vi "Slicing Engine.vi"(7 "System Parameters":T1={"Optical Parameters"={"Obj. Focal Length [mm]"=0.0, "Scan Lens EFL[mm]"=0.0, "Tube Lens EFL[mm]"=0.0, "Galvo V Range (+/-)"=0.0, "Galvo Max Half Angle [Deg]"=0.0, "Max Galvo Range[%]"=0.0}, "Vibratome"={"Z Bottom [mm]"=0.0, "Pre Cut Dwell [s]"=0.0, "Blade Frequency [RPM]"=0, "Slice Speed [mm/s]"=0.0, "Post Cut Dwell [s]"=0.0, "Ramp Time [s]"=0.0, "Start X [mm]"=0.0, "Start Y [mm]"=0.0, "Slice Length [mm]"=0.0, "Slice Axis"=enum."X Axis", "Controller VISA Ref"="COM4"}, "Table Stages"={"X Stage"={"Position"=0.0, "Is.Enabled?"=FALSE, "Is.Connected?"=FALSE, "Device SN"="45876425", "AccelerationMaximum"=50.0, "VelocityMaximum"=50.0, "Acceleration"=50.0, "Velocity"=50.0, "waitTimeout (ms)"=500000, "Model"=enum."Thorlabs LTS", "Is.Homed?"=FALSE}, "Y Stage"={"Position"=0.0, "Is.Enabled?"=FALSE, "Is.Connected?"=FALSE, "Device SN"="45995820", "AccelerationMaximum"=50.0, "VelocityMaximum"=50.0, "Acceleration"=50.0, "Velocity"=50.0, "waitTimeout (ms)"=500000, "Model"=enum."Thorlabs LTS", "Is.Homed?"=FALSE}, "Z Stage"={"Position"=0.0, "Is.Enabled?"=FALSE, "Is.Connected?"=FALSE, "Device SN"="49103464", "AccelerationMaximum"=10.0, "VelocityMaximum"=5.0, "Acceleration"=10.0, "Velocity"=5.0, "waitTimeout (ms)"=100000, "Model"=enum."None", "Is.Homed?"=FALSE}}, "Imaging Parameter"={"Raster Scan Direction"=enum."Uni Directional", "Pixel Dwell Time [Clock Cycles]"=0, "Flyback Time [Clock Cycles]"=0, "XY Center [um]"={"X"=1.0, "Y"=1.0}, "Pixel Step Size [um]"=0.0, "XY Image Size"=enum."32 x 32", "Custom"=FALSE, "Custom Size"={"X"=1, "Y"=1}, "Line Averages"=1}, "Galvo HW Parameters"={"Analog Out Channel"="GalvoCtrl/ao0,GalvoCtrl/ao1", "Min Voltage"=-10.0, "Max Voltage"=10.0, "Pixel Clock Source"="/GalvoCtrl/PFI0", "Sample Rate"=1000.0, "Line Clock Out Ch"="GalvoCtrl/port0/line0"}, "Alazar parameters"={"Trigger Settings"={"General Trigger Settings"={"Trigger Operation"=0, "Coupling ID"=2, "Range ID"=2, "Delay"=0, "Timeout Ticks"=0, "Mode"=1, "Parameter"=1}, "Trigger Engine 1"={"Trigger Engine"=0, "Source"=2, "Slope"=1, "Level"=140}, "Trigger Engine 2"={"Trigger Engine"=1000, "Source"=2048, "Slope"=2048, "Level"=140}}, "Capture Clock"={"Sample Rate"=100, "Decimation"=0, "Source"=2, "Edge"=0}, "Device ID"={"System ID"=1, "Board ID"=1}, "Ch A Input Control"={"Channel"=1, "Coupling"=2, "Range"=10, "Impedance"=2}, "Ch B Input Control"={"Channel"=2, "Coupling"=2, "Range"=10, "Impedance"=2}, "Acq Settings"={"Window Type"=1, "Record Length"=1440, "Footer"=0, "Offset"=0, "Records Per Buffer"=2048, "Samples per record"=2048, "Records Count (Records/Acq)"=2147483647, "Output Format"=10}}, "Mosaic Paramter"={"X Axis"={"Start [mm]"=0.0, "Steps [pts]"=0.0, "End [mm]"=0.0}, "Y Axis"={"Start [mm]"=0.0, "Steps [pts]"=0.0, "End [mm]"=0.0}, "Scan Pattern"=enum."Uni-directional", "Overlap Options"={"Overlap Type"=enum."No Overlap", "Percent Overlap"=0, "Justify"=enum."Start"}}, "Vibratome Axis"={"Start [mm]"=95.8, "thick[um]"=2.1, "#slices"=111}} {"Alazar parameters"."Acq Settings"."Output Format" items=["U16_LOG"=1, "U16_AMP2"=257]; "Alazar parameters"."Acq Settings"."Window Type" items=["DSP_WINDOW_NONE", "DSP_WINDOW_HANNING", "DSP_WINDOW_HAMMING", "DSP_WINDOW_BLACKMAN", "DSP_WINDOW_BLACKMAN_HARRIS", "DSP_WINDOW_BARTLETT"]; "Alazar parameters"."Acq Settings"."Footer" items=["FOOTER_NONE", "FOOTER_NPT"]; "Alazar parameters"."Ch B Input Control"."Channel" items=["A"=1, "B"=2, "C"=4, "D"=8]; "Alazar parameters"."Ch B Input Control"."Coupling" items=["AC"=1, "DC"=2]; "Alazar parameters"."Ch B Input Control"."Range" items=["20 mV"=1, "40 mV"=2, "50 mV"=3, "80 mV"=4, "100 mV"=5, "200 mV"=6, "400 mV"=7, "500 mV"=8, "800 mV"=9, "1 V"=10, "1.25 V"=33, "2 V"=11, "4 V"=12, "5 V"=13, "8 V"=14, "10 V"=15, "20 V"=16]; "Alazar parameters"."Ch B Input Control"."Impedance" items=["1 MOhm"=1, "50 Ohm"=2, ""=0]; "Alazar parameters"."Ch A Input Control"."Channel" items=["A"=1, "B"=2, "C"=4, "D"=8]; "Alazar parameters"."Ch A Input Control"."Coupling" items=["AC"=1, "DC"=2]; "Alazar parameters"."Ch A Input Control"."Range" items=["20 mV"=1, "40 mV"=2, "50 mV"=3, "80 mV"=4, "100 mV"=5, "200 mV"=6, "400 mV"=7, "500 mV"=8, "800 mV"=9, "1 V"=10, "1.25 V"=33, "2 V"=11, "4 V"=12, "5 V"=13, "8 V"=14, "10 V"=15, "20 V"=16]; "Alazar parameters"."Ch A Input Control"."Impedance" items=["1 MOhm"=1, "50 Ohm"=2, ""=0]; "Alazar parameters"."Capture Clock"."Edge" items=["Rising", "Falling"]; "Alazar parameters"."Capture Clock"."Source" items=["Internal"=1, "Fast External"=2, "Medium External"=3, "Slow External"=4, "External AC"=5, "External DC"=6, "External 10MHz"=7]; "Alazar parameters"."Trigger Settings"."General Trigger Settings"."Trigger Operation" items=["J", "K", "J OR K", "J AND K", "J XOR K", "J AND NOT K", "NOT J AND K"]; "Alazar parameters"."Trigger Settings"."General Trigger Settings"."Coupling ID" items=["AC"=1, "DC"=2]; "Alazar parameters"."Trigger Settings"."General Trigger Settings"."Range ID" items=["5 V", "1 V", "TTL"]; "Alazar parameters"."Trigger Settings"."Trigger Engine 1"."Trigger Engine" items=["J", "K"]; "Alazar parameters"."Trigger Settings"."Trigger Engine 1"."Source" items=["A", "B", "External", "Disable", "C", "D"]; "Alazar parameters"."Trigger Settings"."Trigger Engine 1"."Slope" items=["Positive"=1, "Negative"=2]; "Alazar parameters"."Trigger Settings"."Trigger Engine 2"."Trigger Engine" items=["J", "K"]; "Alazar parameters"."Trigger Settings"."Trigger Engine 2"."Source" items=["A", "B", "External", "Disable", "C", "D"]; "Alazar parameters"."Trigger Settings"."Trigger Engine 2"."Slope" items=["Positive"=1, "Negative"=2]; "Imaging Parameter"."Line Averages" min=1 max=30 step=1; "Imaging Parameter"."Flyback Time [Clock Cycles]" max=10 step=1; "Imaging Parameter"."Pixel Step Size [um]" min=0.0 max=10.0 step=0.01; "Imaging Parameter"."Custom Size"."Y" min=1 max=30 step=1; "Imaging Parameter"."Custom Size"."X" min=1 max=30 step=1; "Imaging Parameter"."XY Center [um]"."Y" min=1.0 max=30.0 step=1.0; "Imaging Parameter"."XY Center [um]"."X" min=1.0 max=30.0 step=1.0; "Imaging Parameter"."Pixel Dwell Time [Clock Cycles]" max=10 step=1}, 8 "error in (no error)":errorcluster, 10 "Action":string="Init", 11 "Last Slice?":bool) -> (0 "error out":errorcluster)   [LabVIEW 2018]
uses:
  Controls/System Parameters.ctl
  Controls/Optical Parameters.ctl
  Controls/Vibratome Parameters.ctl
  Controls/Translation Stage Parameters.ctl
  Hardware Mfg/Thorlabs Translation Stages/Controls/Translation Stage Cluster.ctl
  Controls/Translation Stage Types.ctl
  Controls/Imaging Parameters.ctl
  Controls/Scan Direction.ctl
  type defines/Alazar parameters.ctl
  Hardware Mfg/AlazarTech SDK/Controls/General Trigger Settings.ctl
  Hardware Mfg/AlazarTech SDK/Controls/Trigger Engine Controls.ctl
  Hardware Mfg/AlazarTech SDK/Controls/Clock Controls.ctl
  Hardware Mfg/AlazarTech SDK/Controls/Alazar Device ID.ctl
  Hardware Mfg/AlazarTech SDK/Controls/Channel Input Controls.ctl
  Hardware Mfg/AlazarTech SDK/Controls/Alazar Acquisition Settings.ctl
  Controls/Queue Manager Actions.ctl
  Controls/QueueNames.ctl
  Hardware Mfg/Thorlabs Translation Stages/Controls/Motion Translation Module Control.ctl
  Controls/Set Get Controls.ctl
panel:
  # "X"
  # "X"
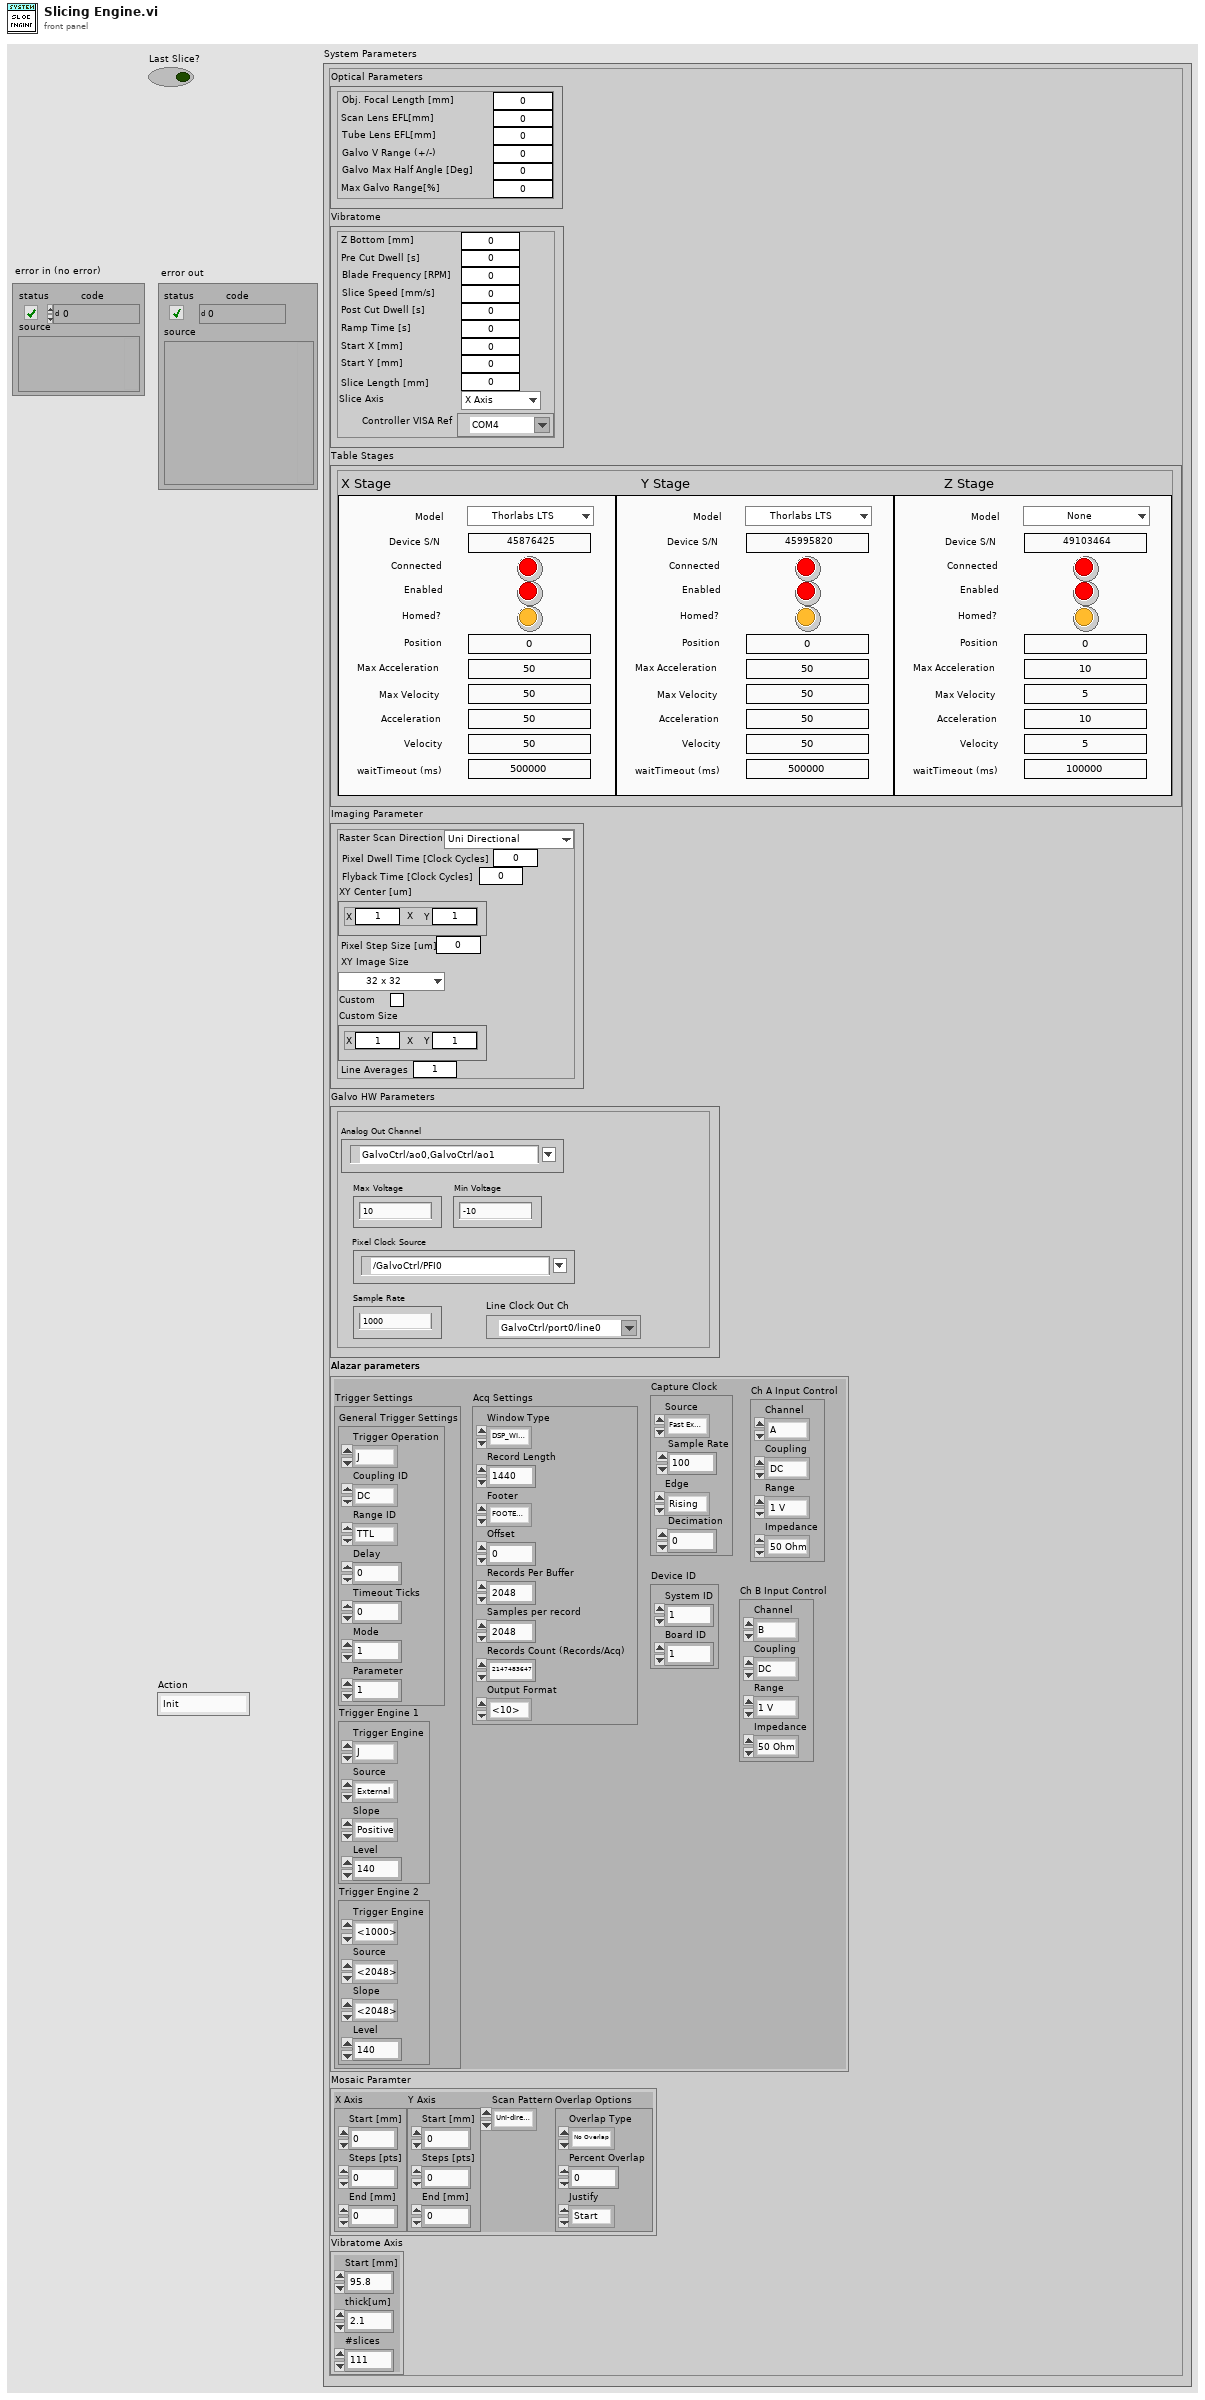
[diagram p1: front panel]
types:
  T1 = typedef "System Parameters.ctl" = cluster{"Optical Parameters":T2, "Vibratome":T3, "Table Stages":T4, "Imaging Parameter":T7, "Galvo HW Parameters":cluster{"Analog Out Channel":tag, "Min Voltage":dbl, "Max Voltage":dbl, "Pixel Clock Source":tag, "Sample Rate":dbl, "Line Clock Out Ch":tag}, "Alazar parameters":T9, "Mosaic Paramter":cluster{"X Axis":cluster{"Start [mm]":dbl, "Steps [pts]":dbl, "End [mm]":dbl}, "Y Axis":cluster{"Start [mm]":dbl, "Steps [pts]":dbl, "End [mm]":dbl}, "Scan Pattern":enum16{"Uni-directional", "Bi-Directional", "Spiral Out", "Spiral In"}, "Overlap Options":cluster{"Overlap Type":enum16{"No Overlap", "X Only", "Y Only", "X and Y"}, "Percent Overlap":u8, "Justify":enum16{"Start", "Center", "End"}}}, "Vibratome Axis":cluster{"Start [mm]":dbl, "thick[um]":dbl, "#slices":u16}}
  T2 = typedef "Optical Parameters.ctl" = cluster{"Obj. Focal Length [mm]":dbl, "Scan Lens EFL[mm]":dbl, "Tube Lens EFL[mm]":dbl, "Galvo V Range (+/-)":dbl, "Galvo Max Half Angle [Deg]":dbl, "Max Galvo Range[%]":dbl}
  T3 = typedef "Vibratome Parameters.ctl" = cluster{"Z Bottom [mm]":dbl, "Pre Cut Dwell [s]":dbl, "Blade Frequency [RPM]":u16, "Slice Speed [mm/s]":dbl, "Post Cut Dwell [s]":dbl, "Ramp Time [s]":dbl, "Start X [mm]":dbl, "Start Y [mm]":dbl, "Slice Length [mm]":dbl, "Slice Axis":enum16{"X Axis", "Y Axis", "Z Axis"}, "Controller VISA Ref":refnum<visa-resource-name>}
  T4 = typedef "Translation Stage Parameters.ctl" = cluster{"X Stage":T5, "Y Stage":T5, "Z Stage":T5}
  T5 = typedef "Translation Stage Cluster.ctl" = cluster{"Position":dbl, "Is.Enabled?":bool, "Is.Connected?":bool, "Device SN":string, "AccelerationMaximum":dbl, "VelocityMaximum":dbl, "Acceleration":dbl, "Velocity":dbl, "waitTimeout (ms)":i32, "Model":T6, "Is.Homed?":bool}
  T6 = typedef "Translation Stage Types.ctl" = enum16{"None", "Thorlabs LTS", "Thorlabs MLJ"}
  T7 = typedef "Imaging Parameters.ctl" = cluster{"Raster Scan Direction":T8, "Pixel Dwell Time [Clock Cycles]":u16, "Flyback Time [Clock Cycles]":u16, "XY Center [um]":cluster{"X":dbl, "Y":dbl}, "Pixel Step Size [um]":dbl, "XY Image Size":enum16{"32 x 32", "64 x 64", "128 x 128", "256 x 256", "512 x 512", "1024 x 1024", "2048 x 2048"}, "Custom":bool, "Custom Size":cluster{"X":u16, "Y":u16}, "Line Averages":u8}
  T8 = typedef "Scan Direction.ctl" = enum16{"Uni Directional", "Bi Directional", "None"}
  T9 = typedef "Alazar parameters.ctl" = cluster{"Trigger Settings":cluster{"General Trigger Settings":T10, "Trigger Engine 1":T11, "Trigger Engine 2":T11}, "Capture Clock":T12, "Device ID":T13, "Ch A Input Control":T14, "Ch B Input Control":T14, "Acq Settings":T15}
  T10 = typedef "General Trigger Settings.ctl" = cluster{"Trigger Operation":u32, "Coupling ID":u32, "Range ID":u32, "Delay":u32, "Timeout Ticks":u32, "Mode":u32, "Parameter":u32}
  T11 = typedef "Trigger Engine Controls.ctl" = cluster{"Trigger Engine":u32, "Source":u32, "Slope":u32, "Level":u32}
  T12 = typedef "Clock Controls.ctl" = cluster{"Sample Rate":u32, "Decimation":u32, "Source":u32, "Edge":u32}
  T13 = typedef "Alazar Device ID.ctl" = cluster{"System ID":u32, "Board ID":u32}
  T14 = typedef "Channel Input Controls.ctl" = cluster{"Channel":u8, "Coupling":u32, "Range":u32, "Impedance":u32}
  T15 = typedef "Alazar Acquisition Settings.ctl" = cluster{"Window Type":u32, "Record Length":u32, "Footer":u32, "Offset":u32, "Records Per Buffer":u32, "Samples per record":u32, "Records Count (Records/Acq)":u32, "Output Format":u32}
  T16 = typedef "QueueNames.ctl" = enum16{"Main GUI", "Main Scan Processor", "Main Processing", "Main Saving", "Main Display", "Main Table Stage GUI", "Main Table Stage Proc.", "Scan Engine", "Vibratome GUI", "Vibratome Processor", "Slice Engine"}
  T17 = typedef "Queue Manager Actions.ctl" = enum16{"Init", "Enqueue", "Enqueue All", "Preview Queue", "Dequeue", "Get Status", "Flush Queue", "Flush All Queues", "Release All Queues", "Release Queue", "Enqueue at Opposite End"}
  T18 = typedef "Set Get Controls.ctl" = enum16{"Set", "Get"}
  T19 = typedef "Motion Translation Module Control.ctl" = enum16{"Init", "Home", "Status", "Velocity/Accel", "Position", "Jog", "Stop", "Uninit", "Enable", "Disable"}
  T20 = enum16{"Set Configuration", "Get Configuration", "Enable Motor", "Disable Motor", "Get Status", "Open Session", "Close Session", "Set Limits", "Get Limits"}
  T21 = cluster{"Source for Velocity":enum16{"Interface", "Voltage (AI)", "PWM (AI)", "Current Target (AI)", "Current Target w/ Preset (AI)"}, "Mode":enum16{"Continuous", "Stepper Motor", "Analog Position Ctrl", "Encoder"}, "Target Velocity [RPM]":i16}
  T22 = typedef "MessagePacket.ctl" = cluster{"Message":string, "Parameter":variant}
  T23 = typedef "Translation Stage Quick Status.ctl" = cluster{"Is.Enabled?":bool, "Is.Connected?":bool, "Is.Homed?":bool}
  T24 = enum16{"Left Button", "Center Button", "Right Button", "Window Close"}
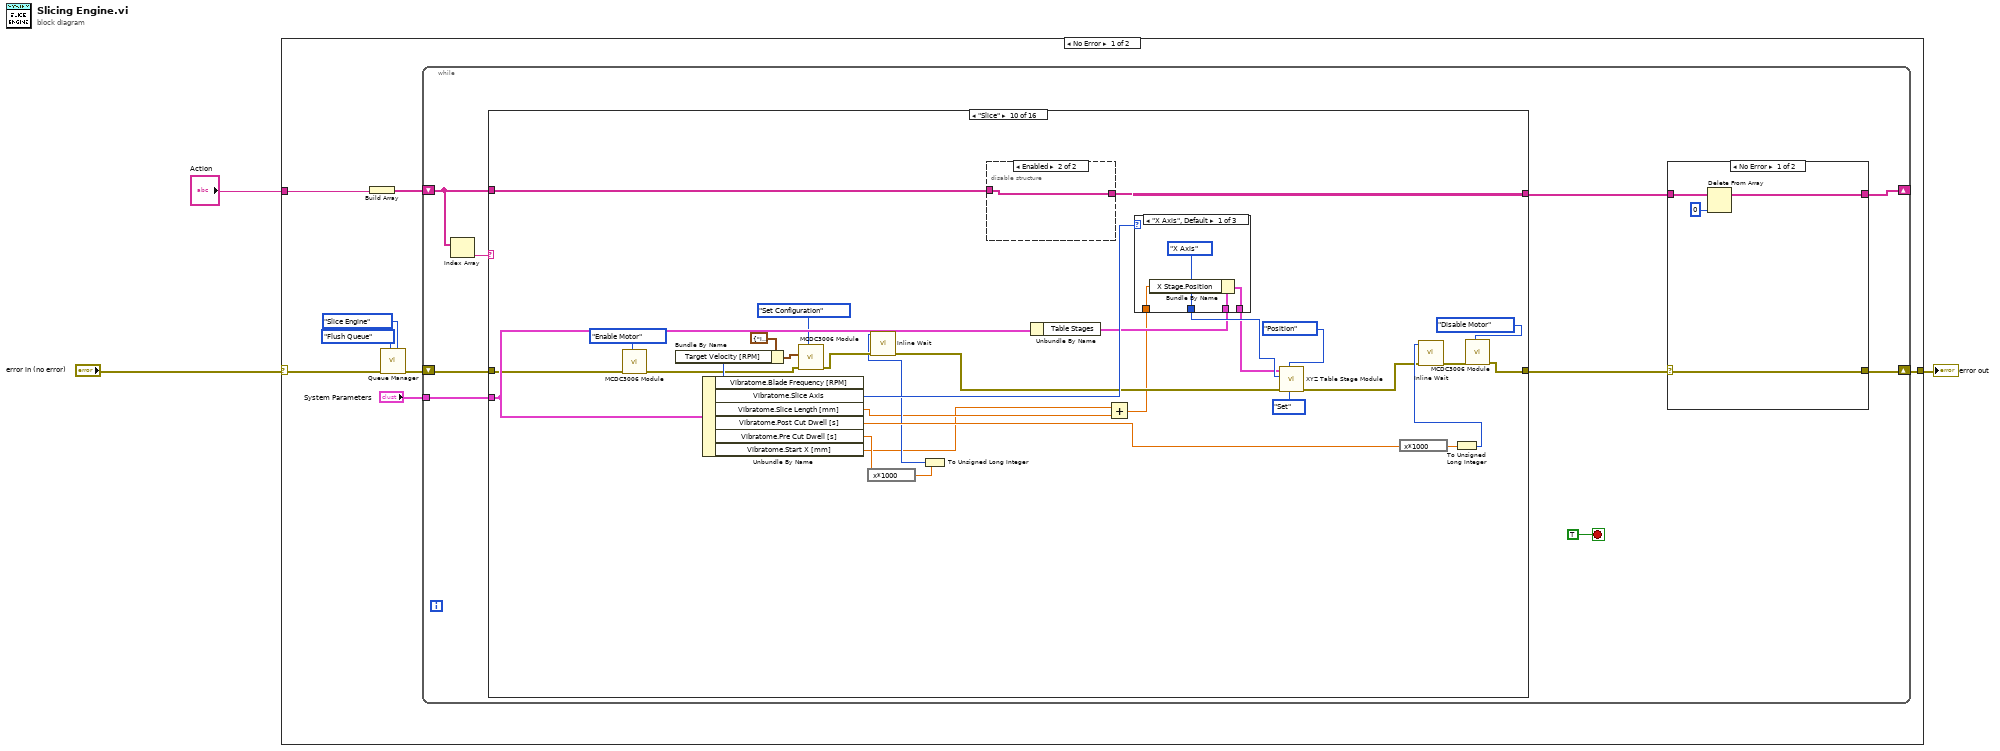
[diagram p0: block diagram]
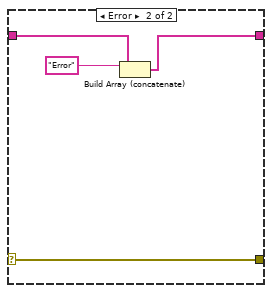
[diagram p2: hidden frame]
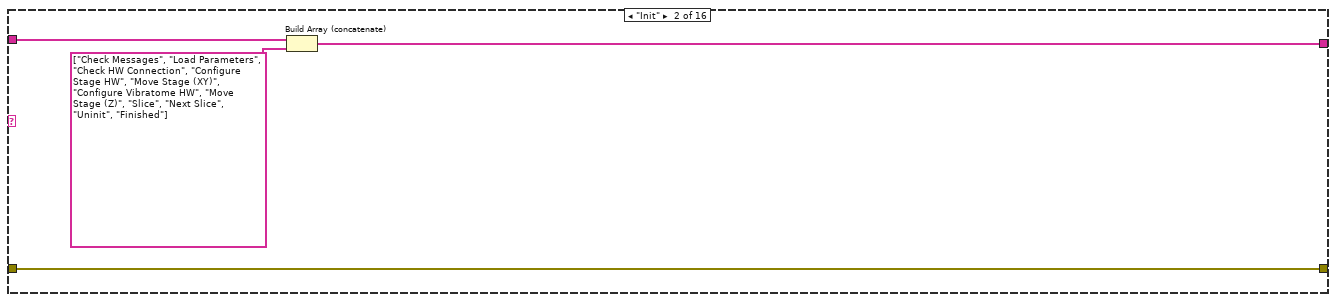
[diagram p4: hidden frame]
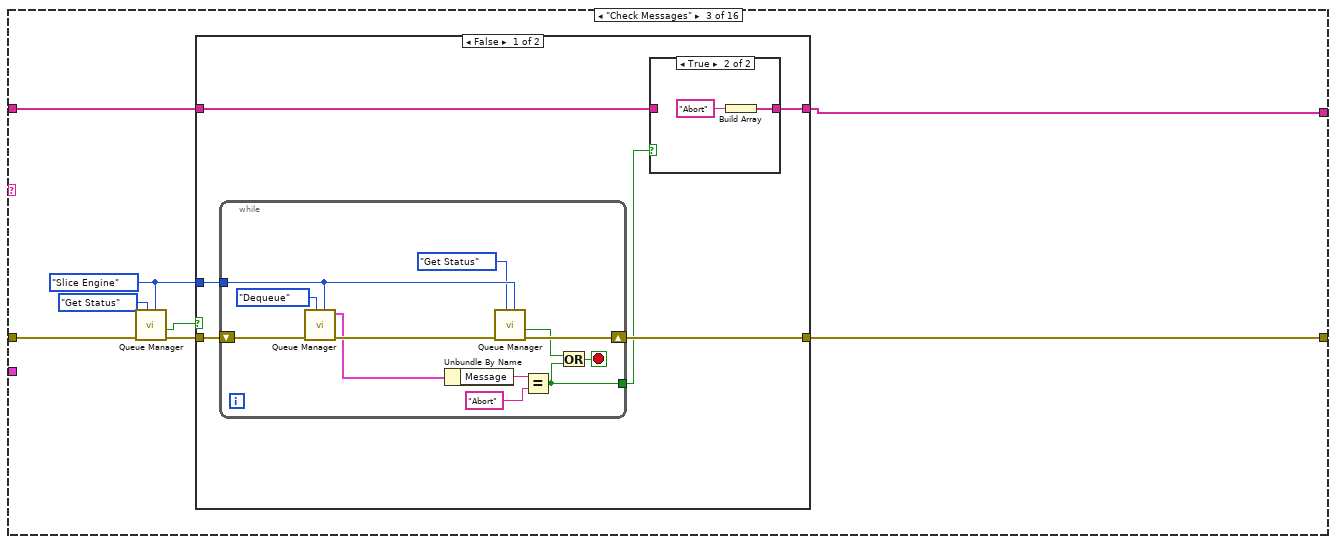
[diagram p5: hidden frame]
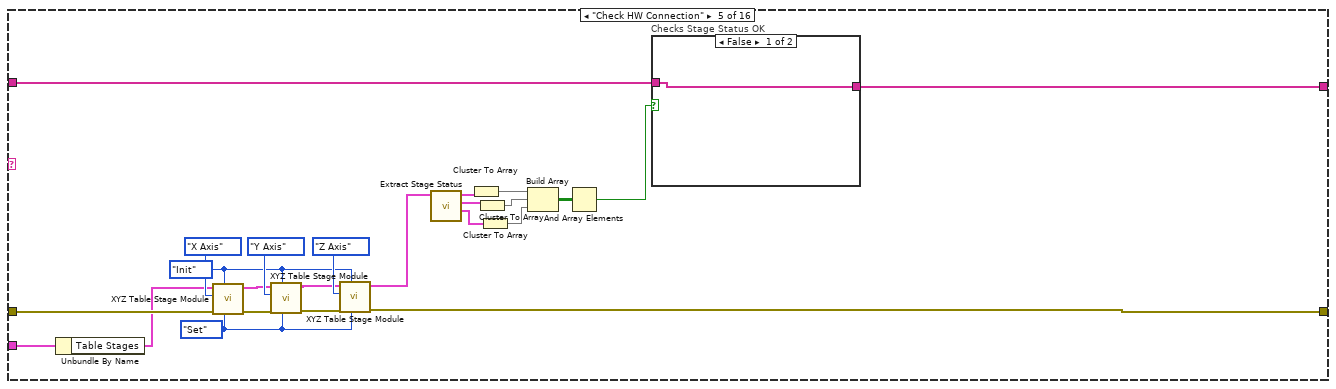
[diagram p9: hidden frame]
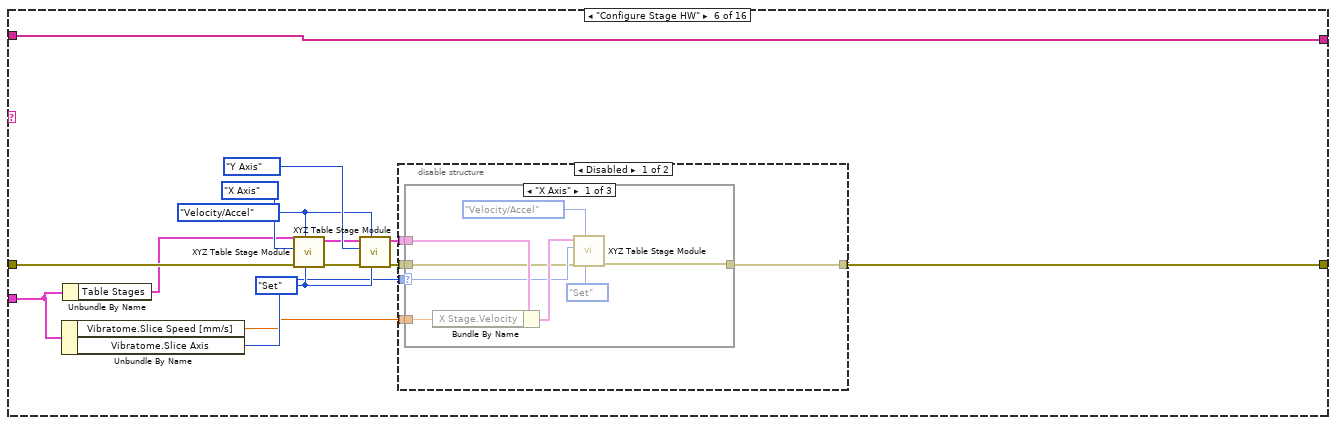
[diagram p11: hidden frame]
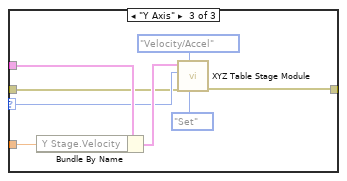
[diagram p13: hidden frame]
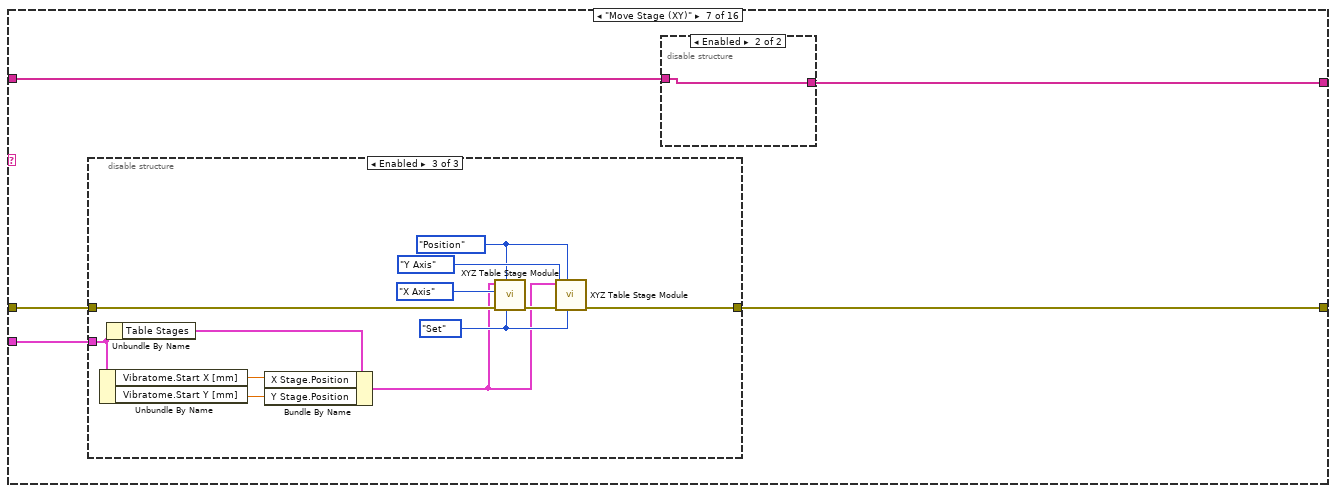
[diagram p15: hidden frame]
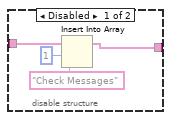
[diagram p16: hidden frame]
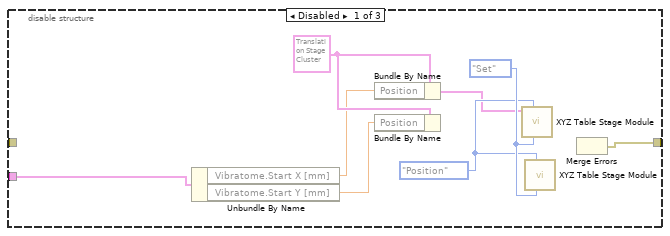
[diagram p17: hidden frame]
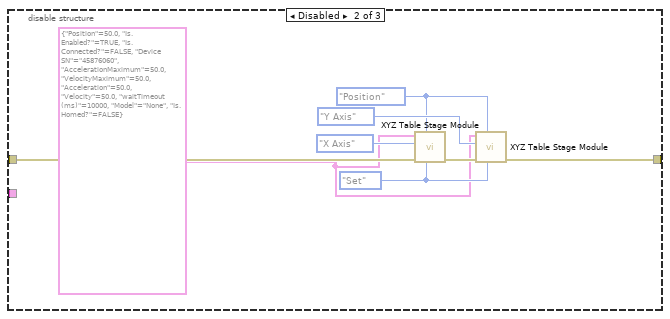
[diagram p18: hidden frame]
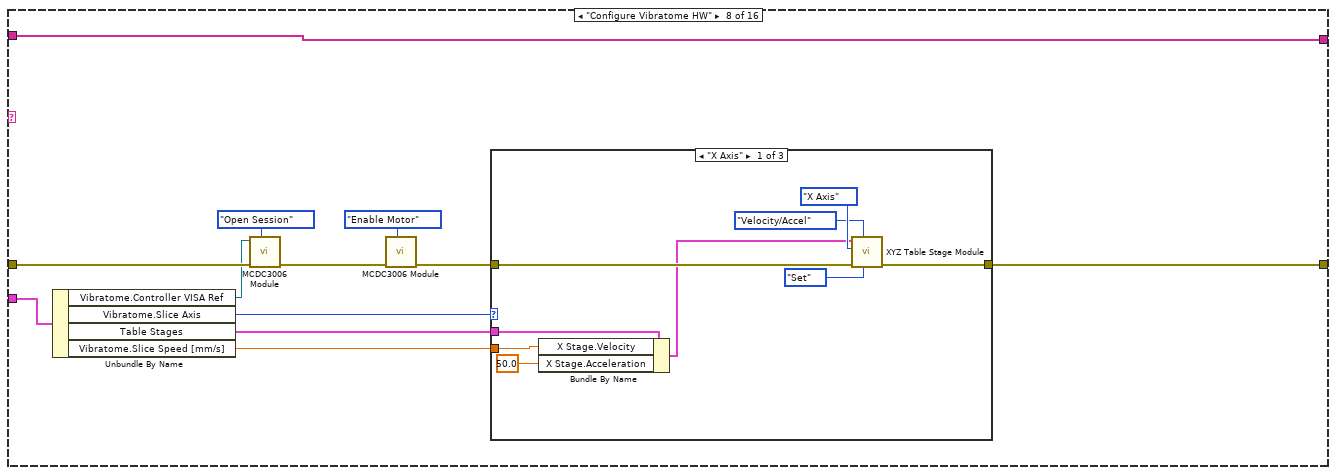
[diagram p19: hidden frame]
diagram:
  n1 = case shown="No Error" "error in (no error)" {
    selector: "error in (no error)" -> [w5 w422]
    tunnel: [w7 w422] -> w2
    tunnel: "Action" -> [w4 _]
    frame No Error {
      n2 = Build Array(w4) -> (w8:string[])
      n3 = call "Queue Manager.vi"("Queue Name"=QueueNames."Slice Engine", "Action"=Queue_Manager_Actions."Flush Queue", "Error In"=w5) -> ("Error Out"=w10:errorcluster)  [unwired: 4 in, 4 out]
      n4 = while {
        shift-right: [w15] -> _
        shift-left: w8 -> [w14]
        shift-right: [w17] -> w7
        shift-left: w10 -> [w20]
        tunnel: "System Parameters" -> [w13]
        stop <- TRUE stop-if-true
        n5 = Index Array(array=w14) -> (element=w19:string)  [unwired: 1 in]
        n6 = case shown="\"Slice\"" w19 {
          tunnel: w20 -> [w29 w31 w42 w66 w91 w107 w134 w179 w202 w247 w272 w298 w312 w316 w345 w420]
          tunnel: w14 -> [w30 w34 w36 w67 w69 w108 w136 w181 w205 w258 w273 w301 w309 w314 w346 w421]
          tunnel: [w30 w33 w35 w67 w70 w108 w135 w181 w204 w257 w273 w300 w310 w313 w346 w421] -> w16
          tunnel: [w29 w31 w37 w66 w89 w94 w133 w173 w203 w241 w274 w298 w312 w317 w343 w419] -> w18
          tunnel: w13 -> [_ _ _ _ w90 w106 w132 w180 w201 w256 w275 _ _ _ w344 _]
          frame "Unknown", Default {
          }
          frame "Init" {
            n7 = Build Array (concatenate)(w34, string[] ["Check Messages", "Load Parameters", "Check HW Connection", "Configure Stage HW", "Move Stage (XY)", "Configure Vibratome HW", "Move Stage (Z)", "Slice", "Next Slice", "Uninit", "Finished"]) -> (w33:string[])
          }
          frame "Check Messages" {
            w38 = QueueNames."Slice Engine" ("Queue Name")
            n8 = call "Queue Manager.vi"("Queue Name"=w38, "Action"=Queue_Manager_Actions."Get Status", "Error In"=w42) -> ("Error Out"=w39:errorcluster, "Empty?"=w40:bool)  [unwired: 4 in, 3 out]
            n9 = case shown="False" w40 {
              tunnel: w39 -> [w48 w64]
              tunnel: w38 -> [w47 _]
              tunnel: [w46 w64] -> w37
              tunnel: w36 -> [w44 w65]
              tunnel: [w43 w65] -> w35
              frame False {
                n10 = while {
                  tunnel: w47 -> [w59]
                  shift-right: [w60] -> w46
                  shift-left: w48 -> [w63]
                  tunnel: [w52] -> w45
                  stop <- w53 stop-if-true
                  n11 = call "Queue Manager.vi"("Queue Name"=w59, "Action"=Queue_Manager_Actions."Dequeue", "Error In"=w63) -> ("Error Out"=w61:errorcluster, "Message Packet [Out]"=w57:T22)  [unwired: 4 in, 3 out]
                  n12 = Unbundle By Name(w57) -> ("Message"=w56:string)
                  n13 = call "Queue Manager.vi"("Queue Name"=w59, "Action"=Queue_Manager_Actions."Get Status", "Error In"=w61) -> ("Error Out"=w60:errorcluster, "Empty?"=w54:bool)  [unwired: 4 in, 3 out]
                  n14 = Equal?(x=w56, y="Abort") -> (x = y?=w52:bool)
                  n15 = Or(x=w54, y=w52) -> (x .or. y?=w53:bool)
                }
                n16 = case shown="True" w45 {
                  tunnel: w44 -> [w49 _]
                  tunnel: [w49 w50] -> w43
                  frame False {
                  }
                  frame True {
                    n17 = Build Array("Abort") -> (w50:string[])
                  }
                }
              }
              frame True {
              }
            }
          }
          frame "Load Parameters" {
          }
          frame "Check HW Connection" {
            w82 = Set_Get_Controls."Set" ("Set/Get")
            w83 = Motion_Translation_Module_Control."Init" ("Action")
            n18 = Unbundle By Name(w90) -> ("Table Stages"=w81:T4)
            n19 = call "XYZ Table Stage Module.vi"("Set/Get"=w82, "Action"=w83, "Error In"=w91, "Axis"=enum16{"X Axis", "Y Axis", "Z Axis"}."X Axis", "Table Stages"=w81) -> ("Error Out"=w88:errorcluster, "Table Stages [out]"=w80:T4)  [unwired: 5 in]
            n20 = call "XYZ Table Stage Module.vi"("Set/Get"=w82, "Action"=w83, "Error In"=w88, "Axis"=enum16{"X Axis", "Y Axis", "Z Axis"}."Y Axis", "Table Stages"=w80) -> ("Error Out"=w87:errorcluster, "Table Stages [out]"=w79:T4)  [unwired: 5 in]
            n21 = call "XYZ Table Stage Module.vi"("Set/Get"=w82, "Action"=w83, "Error In"=w87, "Axis"=enum16{"X Axis", "Y Axis", "Z Axis"}."Z Axis", "Table Stages"=w79) -> ("Error Out"=w89:errorcluster, "Table Stages [out]"=w78:T4)  [unwired: 5 in]
            n22 = call "Extract Stage Status.vi"("Table Stages"=w78) -> ("Z Stage"=w75:T23, "Y Stage"=w76:T23, "X Stage"=w77:T23)  [unwired: 8 in]
            n23 = Cluster To Array(cluster=w77) -> (array=w74:bool[])
            n24 = Cluster To Array(cluster=w76) -> (array=w73:bool[])
            n25 = Cluster To Array(cluster=w75) -> (array=w72:bool[])
            n26 = Build Array(w74, w73, w72) -> (w71:bool[][])
            n27 = And Array Elements(Boolean array=w71) -> (logical AND=w68:bool)
            n28 = case "Checks Stage Status OK" shown="False" w68 {
              tunnel: [w92 w93] -> w70
              tunnel: w69 -> [w92 w93]
              frame False {
              }
              frame True {
              }
            }
          }
          frame "Configure Stage HW" {
            w101 = Set_Get_Controls."Set" ("Set/Get")
            w102 = Motion_Translation_Module_Control."Velocity/Accel" ("Action")
            n29 = Unbundle By Name(w106) -> ("Vibratome.Slice Speed [mm/s]"=w97:dbl, "Vibratome.Slice Axis"=w98:enum16{"X Axis", "Y Axis", "Z Axis"})
            n30 = Unbundle By Name(w106) -> ("Table Stages"=w99:T4)
            n31 = call "XYZ Table Stage Module.vi"("Set/Get"=w101, "Action"=w102, "Error In"=w107, "Axis"=enum16{"X Axis", "Y Axis", "Z Axis"}."X Axis", "Table Stages"=w99) -> ("Error Out"=w105:errorcluster, "Table Stages [out]"=w100:T4)  [unwired: 5 in]
            n32 = call "XYZ Table Stage Module.vi"("Set/Get"=w101, "Action"=w102, "Error In"=w105, "Axis"=enum16{"X Axis", "Y Axis", "Z Axis"}."Y Axis", "Table Stages"=w100) -> ("Error Out"=w95:errorcluster, "Table Stages [out]"=w96:T4)  [unwired: 5 in]
            n33 = disable-structure shown="Disabled" {
              disable-tunnel: w98 -> [w113 _]
              disable-tunnel: w97 -> [w112 _]
              disable-tunnel: w96 -> [w111 _]
              disable-tunnel: w95 -> [w110 w131]
              disable-tunnel: [w109 w131] -> w94
              frame Disabled {
                n34 = case shown="\"X Axis\"" w113 {
                  selector: w113 -> [w118 _ w127]
                  tunnel: w112 -> [w121 _ w130]
                  tunnel: w111 -> [w120 _ w129]
                  tunnel: w110 -> [w117 w122 w126]
                  tunnel: [w116 w122 w125] -> w109
                  frame "X Axis" {
                    n35 = Bundle By Name(cluster=w120, "X Stage.Velocity"=w121) -> (w119:T4)
                    n36 = call "XYZ Table Stage Module.vi"("Set/Get"=Set_Get_Controls."Set", "Action"=Motion_Translation_Module_Control."Velocity/Accel", "Error In"=w117, "Axis"=w118, "Table Stages"=w119) -> ("Error Out"=w116:errorcluster)  [unwired: 5 in, 1 out]
                  }
                  frame "Z Axis" {
                  }
                  frame "Y Axis" {
                    n37 = Bundle By Name(cluster=w129, "Y Stage.Velocity"=w130) -> (w128:T4)
                    n38 = call "XYZ Table Stage Module.vi"("Set/Get"=Set_Get_Controls."Set", "Action"=Motion_Translation_Module_Control."Velocity/Accel", "Error In"=w126, "Axis"=w127, "Table Stages"=w128) -> ("Error Out"=w125:errorcluster)  [unwired: 5 in, 1 out]
                  }
                }
              }
              frame Enabled {
              }
            }
          }
          frame "Move Stage (XY)" {
            n39 = disable-structure shown="Enabled" {
              disable-tunnel: w134 -> [_ w155 w167]
              disable-tunnel: [w149 w156 w168] -> w133
              disable-tunnel: w132 -> [w147 _ w162]
              frame Disabled {
                w148 = T5 {"Position"=0.0, "Is.Enabled?"=TRUE, "Is.Connected?"=FALSE, "Device SN"="45876060", "AccelerationMaximum"=50.0, "VelocityMaximum"=50.0, "Acceleration"=50.0, "Velocity"=50.0, "waitTimeout (ms)"=10000, "Model"=enum."None", "Is.Homed?"=FALSE} ("Cluster In")
                w143 = Motion_Translation_Module_Control."Position" ("Action")
                w144 = Set_Get_Controls."Set" ("Set/Get")
                n40 = Unbundle By Name(w147) -> ("Vibratome.Start X [mm]"=w146:dbl, "Vibratome.Start Y [mm]"=w145:dbl)
                n41 = Bundle By Name(cluster=w148, "Position"=w146) -> (w142:T5)
                n42 = Bundle By Name(cluster=w148, "Position"=w145) -> ()  [unwired: 1 out]
                n43 = call "XYZ Table Stage Module.vi"("Set/Get"=w144, "Action"=w143, "Table Stages"=w142) -> ()  [unwired: 7 in, 2 out]
                n44 = call "XYZ Table Stage Module.vi"("Set/Get"=w144, "Action"=w143) -> ()  [unwired: 8 in, 2 out]
                n45 = Merge Errors() -> (w149:errorcluster)  [unwired: 2 in]
              }
              frame Disabled {
                w151 = Set_Get_Controls."Set" ("Set/Get")
                w152 = Motion_Translation_Module_Control."Position" ("Action")
                w150 = T5 {"Position"=50.0, "Is.Enabled?"=TRUE, "Is.Connected?"=FALSE, "Device SN"="45876060", "AccelerationMaximum"=50.0, "VelocityMaximum"=50.0, "Acceleration"=50.0, "Velocity"=50.0, "waitTimeout (ms)"=10000, "Model"=enum."None", "Is.Homed?"=FALSE} ("Cluster In")
                n46 = call "XYZ Table Stage Module.vi"("Set/Get"=w151, "Action"=w152, "Error In"=w155, "Axis"=enum16{"X Axis", "Y Axis", "Z Axis"}."X Axis", "Table Stages"=w150) -> ("Error Out"=w157:errorcluster)  [unwired: 5 in, 1 out]
                n47 = call "XYZ Table Stage Module.vi"("Set/Get"=w151, "Action"=w152, "Error In"=w157, "Axis"=enum16{"X Axis", "Y Axis", "Z Axis"}."Y Axis", "Table Stages"=w150) -> ("Error Out"=w156:errorcluster)  [unwired: 5 in, 1 out]
              }
              frame Enabled {
                w163 = Set_Get_Controls."Set" ("Set/Get")
                w164 = Motion_Translation_Module_Control."Position" ("Action")
                n48 = Unbundle By Name(w162) -> ("Vibratome.Start X [mm]"=w160:dbl, "Vibratome.Start Y [mm]"=w159:dbl)
                n49 = Unbundle By Name(w162) -> ("Table Stages"=w161:T4)
                n50 = Bundle By Name(cluster=w161, "X Stage.Position"=w160, "Y Stage.Position"=w159) -> (w158:T4)
                n51 = call "XYZ Table Stage Module.vi"("Set/Get"=w163, "Action"=w164, "Error In"=w167, "Axis"=enum16{"X Axis", "Y Axis", "Z Axis"}."X Axis", "Table Stages"=w158) -> ("Error Out"=w169:errorcluster)  [unwired: 5 in, 1 out]
                n52 = call "XYZ Table Stage Module.vi"("Set/Get"=w163, "Action"=w164, "Error In"=w169, "Axis"=enum16{"X Axis", "Y Axis", "Z Axis"}."Y Axis", "Table Stages"=w158) -> ("Error Out"=w168:errorcluster)  [unwired: 5 in, 1 out]
              }
            }
            n53 = disable-structure shown="Enabled" {
              disable-tunnel: w136 -> [w140 w141]
              disable-tunnel: [w139 w141] -> w135
              frame Disabled {
                n54 = Insert Into Array(array=w140, index=1, new element="Check Messages" ("new element/subarray")) -> (w139:string[])
              }
              frame Enabled {
              }
            }
          }
          frame "Configure Vibratome HW" {
            n55 = Unbundle By Name(w180) -> ("Vibratome.Controller VISA Ref"=w177:refnum<visa-resource-name>, "Vibratome.Slice Axis"=w172:enum16{"X Axis", "Y Axis", "Z Axis"}, "Table Stages"=w170:T4, "Vibratome.Slice Speed [mm/s]"=w171:dbl)
            n56 = call "MCDC3006 Module.vi"("Actions"=T20."Open Session", "Error In"=w179, "VISA resource name"=w177) -> ("Error Out"=w175:errorcluster)  [unwired: 4 in, 4 out]
            n57 = call "MCDC3006 Module.vi"("Actions"=T20."Enable Motor", "Error In"=w175) -> ("Error Out"=w174:errorcluster)  [unwired: 5 in, 4 out]
            n58 = case shown="\"X Axis\"" w172 {
              tunnel: [w190 w191 w200] -> w173
              tunnel: w174 -> [w185 w191 w196]
              tunnel: w171 -> [w186 _ w195]
              tunnel: w170 -> [w183 _ w194]
              frame "X Axis" {
                n59 = Bundle By Name(cluster=w183, "X Stage.Velocity"=w186, "X Stage.Acceleration"=50.0 ("Acceleration")) -> (w182:T4)
                n60 = call "XYZ Table Stage Module.vi"("Set/Get"=Set_Get_Controls."Set", "Action"=Motion_Translation_Module_Control."Velocity/Accel", "Error In"=w185, "Axis"=enum16{"X Axis", "Y Axis", "Z Axis"}."X Axis", "Table Stages"=w182) -> ("Error Out"=w190:errorcluster)  [unwired: 5 in, 1 out]
              }
              frame "Z Axis" {
              }
              frame "Y Axis" {
                n61 = Bundle By Name(cluster=w194, "Y Stage.Velocity"=w195, "Y Stage.Acceleration"=50.0 ("Acceleration")) -> (w192:T4)
                n62 = call "XYZ Table Stage Module.vi"("Set/Get"=Set_Get_Controls."Set", "Action"=Motion_Translation_Module_Control."Velocity/Accel", "Error In"=w196, "Axis"=enum16{"X Axis", "Y Axis", "Z Axis"}."Y Axis", "Table Stages"=w192) -> ("Error Out"=w200:errorcluster)  [unwired: 5 in, 1 out]
              }
            }
          }
          frame "Move Stage (Z)" {
            n63 = disable-structure shown="Disabled" {
              disable-tunnel: [w214 w222] -> w203
              disable-tunnel: w202 -> [w213 w222]
              disable-tunnel: w201 -> [w212 _]
              frame Disabled {
                n64 = Unbundle By Name(w212) -> ("Table Stages"=w211:T4)
                n65 = call "XYZ Table Stage Module.vi"("Set/Get"=Set_Get_Controls."Get", "Action"=Motion_Translation_Module_Control."Position", "Error In"=w213, "Axis"=enum16{"X Axis", "Y Axis", "Z Axis"}."Z Axis", "Table Stages"=w211) -> ("Error Out"=w215:errorcluster, "Table Stages [out]"=w210:T4)  [unwired: 5 in]
                n66 = Unbundle By Name(w210) -> ("Z Stage.Position"=w208:dbl)
                n67 = Add(x=w208, y=0.2) -> (x+y=w206:dbl)
                n68 = Bundle By Name(cluster=w210, "Z Stage.Position"=w206) -> (w209:T4)
                n69 = call "XYZ Table Stage Module.vi"("Set/Get"=Set_Get_Controls."Set", "Action"=Motion_Translation_Module_Control."Position", "Error In"=w215, "Axis"=enum16{"X Axis", "Y Axis", "Z Axis"}."Z Axis", "Table Stages"=w209) -> ("Error Out"=w214:errorcluster)  [unwired: 5 in, 1 out]
              }
              frame Enabled {
              }
            }
            n70 = disable-structure shown="Enabled" {
              disable-tunnel: w205 -> [w226 w227]
              disable-tunnel: [w225 w227] -> w204
              frame Disabled {
                n71 = Insert Into Array(array=w226, index=1, new element="Check Messages" ("new element/subarray")) -> (w225:string[])
              }
              frame Enabled {
              }
            }
          }
          frame "Slice" {
            n72 = call "MCDC3006 Module.vi"("Actions"=T20."Enable Motor", "Error In"=w247) -> ("Error Out"=w246:errorcluster)  [unwired: 5 in, 4 out]
            n73 = Unbundle By Name(w256) -> ("Vibratome.Blade Frequency [RPM]"=w251:u16, "Vibratome.Slice Axis"=w255:enum16{"X Axis", "Y Axis", "Z Axis"}, "Vibratome.Slice Length [mm]"=w235:dbl, "Vibratome.Post Cut Dwell [s]"=w249:dbl, "Vibratome.Pre Cut Dwell [s]"=w245:dbl, "Vibratome.Start X [mm]"=w234:dbl)
            n74 = Bundle By Name(cluster=T21 {"Source for Velocity"=enum."Interface", "Mode"=enum."Continuous", "Target Velocity [RPM]"=0} ("Configuration [In]"), "Target Velocity [RPM]"=w251) -> (w250:T21)
            n75 = call "MCDC3006 Module.vi"("Actions"=T20."Set Configuration", "Error In"=w246, "Configuration [In]"=w250) -> ("Error Out"=w254:errorcluster)  [unwired: 4 in, 4 out]
            n76 = expression code="x*1000"(w245) -> (w244:dbl)
            n77 = To Unsigned Long Integer(number=w244) -> (unsigned 32bit integer=w243:u32)
            n78 = call "Inline Wait.vi"("Error In"=w254, "milliseconds to wait"=w243) -> ("Error Out"=w236:errorcluster)  [unwired: 9 in]
            n79 = disable-structure shown="Enabled" {
              disable-tunnel: w258 -> [w270 w271]
              disable-tunnel: [w269 w271] -> w257
              frame Disabled {
                n80 = Insert Into Array(array=w270, index=1, new element="Check Messages" ("new element/subarray")) -> (w269:string[])
              }
              frame Enabled {
              }
            }
            n81 = Unbundle By Name(w256) -> ("Table Stages"=w231:T4)
            n82 = Add(x=w234, y=w235) -> (x+y=w230:dbl)
            n83 = case shown="\"X Axis\", Default" w255 {
              tunnel: [enum16{"X Axis", "Y Axis", "Z Axis"}."X Axis" ("Axis") _ enum16{"X Axis", "Y Axis", "Z Axis"}."Y Axis" ("Axis")] -> w232
              tunnel: w231 -> [w261 _ w264]
              tunnel: w230 -> [w260 _ w265]
              tunnel: [w259 _ w263] -> w229
              frame "X Axis", Default {
                n84 = Bundle By Name(cluster=w261, "X Stage.Position"=w260) -> (w259:T4)
              }
              frame "Z Axis" {
              }
              frame "Y Axis" {
                n85 = Bundle By Name(cluster=w264, "X Stage.Position"=w265) -> (w263:T4)
              }
            }
            n86 = call "XYZ Table Stage Module.vi"("Set/Get"=Set_Get_Controls."Set", "Action"=Motion_Translation_Module_Control."Position", "Error In"=w236, "Axis"=w232, "Table Stages"=w229) -> ("Error Out"=w233:errorcluster)  [unwired: 5 in, 1 out]
            n87 = expression code="x*1000"(w249) -> (w240:dbl)
            n88 = To Unsigned Long Integer(number=w240) -> (unsigned 32bit integer=w239:u32)
            n89 = call "Inline Wait.vi"("Error In"=w233, "milliseconds to wait"=w239) -> ("Error Out"=w242:errorcluster)  [unwired: 9 in]
            n90 = call "MCDC3006 Module.vi"("Actions"=T20."Disable Motor", "Error In"=w242) -> ("Error Out"=w241:errorcluster)  [unwired: 5 in, 4 out]
          }
          frame "set slice speed" {
            n91 = Unbundle By Name(w275) -> ("Vibratome.Slice Axis"=w278:enum16{"X Axis", "Y Axis", "Z Axis"}, "Table Stages"=w276:T4, "Vibratome.Slice Speed [mm/s]"=w277:dbl)
            n92 = case shown="\"X Axis\"" w278 {
              tunnel: [w287 w288 w297] -> w274
              tunnel: w272 -> [w282 w288 w293]
              tunnel: w277 -> [w283 _ w292]
              tunnel: w276 -> [w280 _ w291]
              frame "X Axis" {
                n93 = Bundle By Name(cluster=w280, "X Stage.Velocity"=w283, "X Stage.Acceleration"=50.0 ("Acceleration")) -> (w279:T4)
                n94 = call "XYZ Table Stage Module.vi"("Set/Get"=Set_Get_Controls."Set", "Action"=Motion_Translation_Module_Control."Velocity/Accel", "Error In"=w282, "Axis"=enum16{"X Axis", "Y Axis", "Z Axis"}."X Axis", "Table Stages"=w279) -> ("Error Out"=w287:errorcluster)  [unwired: 5 in, 1 out]
              }
              frame "Z Axis" {
              }
              frame "Y Axis" {
                n95 = Bundle By Name(cluster=w291, "Y Stage.Velocity"=w292, "Y Stage.Acceleration"=50.0 ("Acceleration")) -> (w289:T4)
                n96 = call "XYZ Table Stage Module.vi"("Set/Get"=Set_Get_Controls."Set", "Action"=Motion_Translation_Module_Control."Velocity/Accel", "Error In"=w293, "Axis"=enum16{"X Axis", "Y Axis", "Z Axis"}."Y Axis", "Table Stages"=w289) -> ("Error Out"=w297:errorcluster)  [unwired: 5 in, 1 out]
              }
            }
          }
          frame "Next Slice" {
            n97 = case shown="False" "Last Slice?" {
              tunnel: w301 -> [w305 w306]
              tunnel: [w304 w306] -> w300
              frame False {
                n98 = Insert Into Array(array=w305, index=1, new element=string[] ["Move Stage (Z)", "set slice speed", "Slice", "Next Slice"]) -> (w304:string[])
              }
              frame True {
              }
            }
          }
          frame "Abort" {
            n99 = Insert Into Array(array=w309, index=1, new element #1="Uninit", new element #2="Finished") -> (w310:string[])
          }
          frame "Error" {
            n100 = control-ref of="This VI"() -> (w327:refnum<vi>)
            n101 = property class="VI"(reference=w327) -> ("Name"=w330:string, "Callers"=w332:string[])  [unwired: 1 in, 2 out]
            n102 = Unbundle(w316) -> ("code"=w326:i32, "source"=w325:string)  [unwired: 1 out]
            n103 = Array To Spreadsheet String(delimiter (Tab)=">", array=w332, 3:"%s" ("format string")) -> (spreadsheet string=w331:string)
            n104 = Format Into String(format string="VI Name: %s\nCallers: %s\nError Code: %d\nError Message: %s", initial string="The following error occurred:\n" ("message"), w330, w331, w326, w325) -> (resulting string=w324:string, error out=w318:errorcluster)  [unwired: 1 in]
            n105 = call <vilib>:"Clear Errors.vi"("error in (no error)"=w318) -> ()  [unwired: 5 in, 2 out]
            n106 = call <vilib>:"Three Button Dialog.vi"("Allow user to close window? (TRUE)"=FALSE, "Window Title (\"\")"="Error" ("Window Title (\"\")"), "Right Button Text (\"Cancel\")"="Abort" ("Right Button Text (\"Cancel\")"), "Center Button Text (\"No\")"="Retry" ("Center Button Text (\"No\")"), "Left Button Text (\"Yes\")"="Continue" ("Left Button Text (\"Yes\")"), "message"=w324) -> ("Which Button?"=w315:T24)  [unwired: 5 in]
            n107 = case shown="\"Right Button\"" w315 {
              tunnel: w314 -> [w337 w341 w342]
              tunnel: [w336 w340 w342] -> w313
              frame "Left Button", Default {
                # "Continue"
                n108 = Delete From Array(array=w337, index=0) -> (array with subset deleted=w336:string[])  [unwired: 1 in, 1 out]
              }
              frame "Right Button" {
                # "Abort"
                n109 = Insert Into Array(array=w341, index=1, new element="Abort") -> (w340:string[])
              }
              frame "Center Button" {
                # "Retry"
              }
            }
            n110 = call <vilib>:"Clear Errors.vi"("error in (no error)"=w316) -> ("error out"=w317:errorcluster)  [unwired: 5 in, 1 out]
          }
          frame "Uninit" {
            n111 = disable-structure shown="Enabled" {
              disable-tunnel: w345 -> [w350 w417]
              disable-tunnel: w344 -> [w349 _]
              disable-tunnel: [w348 w410] -> w343
              frame Enabled {
                n112 = for {
                  N: 4 -> [_]
                  tunnel: [w356] -> w351 mode=indexing
                  tunnel: Motion_Translation_Module_Control."Uninit" ("Action") -> [w355]
                  tunnel: w350 -> [w354]
                  tunnel: w349 -> [w353]
                  i -> [w357]
                  n113 = case shown="0, Default" w357 {
                    tunnel: [w363 w377 w391 w403] -> w356
                    tunnel: w354 -> [w362 w376 w390 w404]
                    tunnel: w355 -> [w361 w375 w389 _]
                    tunnel: w353 -> [w360 w374 w388 _]
                    frame 0, Default {
                      # "X Stage"
                      n114 = Unbundle By Name(w360) -> ("Table Stages.X Stage.Model"=w359:T6, "Table Stages.X Stage.Device SN"=w358:string)
                      n115 = case shown="\"Thorlabs LTS\"" w359 {
                        tunnel: [w364 w371] -> w363
                        tunnel: w362 -> [w364 w370]
                        tunnel: w361 -> [_ w369]
                        tunnel: w358 -> [_ w367]
                        frame "None", Default {
                        }
                        frame "Thorlabs LTS" {
                          n116 = Bundle By Name(cluster=T5 {"Position"=0.0, "Is.Enabled?"=TRUE, "Is.Connected?"=FALSE, "Device SN"="45876539", "AccelerationMaximum"=0.0, "VelocityMaximum"=0.0, "Acceleration"=0.0, "Velocity"=0.0, "waitTimeout (ms)"=0, "Model"=enum."Thorlabs LTS", "Is.Homed?"=FALSE} ("Cluster In"), "Device SN"=w367) -> (w366:T5)
                          n117 = call "Thorlabs LTS - X Stage Module.vi"("Set/Get"=Set_Get_Controls."Set", "Error In"=w370, "Action"=w369, "Cluster In"=w366) -> ("Error Out"=w371:errorcluster)  [unwired: 6 in, 1 out]
                        }
                      }
                    }
                    frame 1 {
                      # "Y Stage"
                      n118 = Unbundle By Name(w374) -> ("Table Stages.Y Stage.Model"=w373:T6, "Table Stages.Y Stage.Device SN"=w372:string)
                      n119 = case shown="\"Thorlabs LTS\"" w373 {
                        tunnel: [w378 w385] -> w377
                        tunnel: w376 -> [w378 w384]
                        tunnel: w375 -> [_ w383]
                        tunnel: w372 -> [_ w381]
                        frame "None", Default {
                        }
                        frame "Thorlabs LTS" {
                          n120 = Bundle By Name(cluster=T5 {"Position"=0.0, "Is.Enabled?"=TRUE, "Is.Connected?"=FALSE, "Device SN"="45876539", "AccelerationMaximum"=0.0, "VelocityMaximum"=0.0, "Acceleration"=0.0, "Velocity"=0.0, "waitTimeout (ms)"=0, "Model"=enum."Thorlabs LTS", "Is.Homed?"=FALSE} ("Cluster In"), "Device SN"=w381) -> (w380:T5)
                          n121 = call "Thorlabs LTS - Y Stage Module.vi"("Set/Get"=Set_Get_Controls."Set", "Error In"=w384, "Action"=w383, "Cluster In"=w380) -> ("Error Out"=w385:errorcluster)  [unwired: 6 in, 1 out]
                        }
                      }
                    }
                    frame 2 {
                      # "Z Stage"
                      n122 = Unbundle By Name(w388) -> ("Table Stages.Z Stage.Model"=w387:T6, "Table Stages.Z Stage.Device SN"=w386:string)
                      n123 = case shown="\"Thorlabs MLJ\"" w387 {
                        tunnel: [w392 w399] -> w391
                        tunnel: w390 -> [w392 w398]
                        tunnel: w389 -> [_ w397]
                        tunnel: w386 -> [_ w395]
                        frame "None", Default {
                        }
                        frame "Thorlabs MLJ" {
                          n124 = Bundle By Name(cluster=T5 {"Position"=0.0, "Is.Enabled?"=TRUE, "Is.Connected?"=FALSE, "Device SN"="45876539", "AccelerationMaximum"=0.0, "VelocityMaximum"=0.0, "Acceleration"=0.0, "Velocity"=0.0, "waitTimeout (ms)"=0, "Model"=enum."Thorlabs MLJ", "Is.Homed?"=FALSE} ("Cluster In"), "Device SN"=w395) -> (w394:T5)
                          n125 = call "Thorlabs MLJ - Z Stage Module.vi"("Set/Get"=Set_Get_Controls."Set", "Error In"=w398, "Action"=w397, "Cluster In"=w394) -> ("Error Out"=w399:errorcluster)  [unwired: 6 in, 1 out]
                        }
                      }
                    }
                    frame 3 {
                      # "Vibratome Motor"
                      n126 = call "MCDC3006 Module.vi"("Actions"=T20."Disable Motor", "Error In"=w404) -> ("Error Out"=w401:errorcluster)  [unwired: 5 in, 4 out]
                      n127 = call "MCDC3006 Module.vi"("Actions"=T20."Close Session", "Error In"=w401) -> ("Error Out"=w403:errorcluster)  [unwired: 5 in, 4 out]
                    }
                  }
                }
                n128 = Merge Errors(w351) -> (w348:errorcluster)
              }
              frame Disabled {
                w405 = Set_Get_Controls."Set" ("Set/Get")
                w409 = Motion_Translation_Module_Control."Uninit" ("Action")
                n129 = call "XYZ Table Stage Module.vi"("Set/Get"=w405, "Action"=w409, "Error In"=w417, "Axis"=enum16{"X Axis", "Y Axis", "Z Axis"}."X Axis") -> ("Error Out"=w416:errorcluster)  [unwired: 6 in, 1 out]
                n130 = call "XYZ Table Stage Module.vi"("Set/Get"=w405, "Action"=w409, "Error In"=w416, "Axis"=enum16{"X Axis", "Y Axis", "Z Axis"}."Y Axis") -> ("Error Out"=w415:errorcluster)  [unwired: 6 in, 1 out]
                n131 = call "XYZ Table Stage Module.vi"("Set/Get"=w405, "Action"=w409, "Error In"=w415, "Axis"=enum16{"X Axis", "Y Axis", "Z Axis"}."Z Axis") -> ("Error Out"=w412:errorcluster)  [unwired: 6 in, 1 out]
                n132 = call "MCDC3006 Module.vi"("Actions"=T20."Disable Motor", "Error In"=w412) -> ("Error Out"=w411:errorcluster)  [unwired: 5 in, 4 out]
                n133 = call "MCDC3006 Module.vi"("Actions"=T20."Close Session", "Error In"=w411) -> ("Error Out"=w410:errorcluster)  [unwired: 5 in, 4 out]
              }
            }
          }
          frame "Finished" {
            n134 = call "Inline Wait.vi"("Error In"=w420, "milliseconds to wait"=u32 1000) -> ("Error Out"=w419:errorcluster)  [unwired: 9 in]
          }
        }
        n135 = case shown="No Error" w18 {
          selector: w18 -> [w24 w25]
          tunnel: [w24 w25] -> w17
          tunnel: w16 -> [w23 w28]
          tunnel: [w22 w26] -> w15
          frame No Error {
            n136 = Delete From Array(array=w23, index=0) -> (array with subset deleted=w22:string[])  [unwired: 1 in, 1 out]
          }
          frame Error {
            n137 = Build Array (concatenate)("Error", w28) -> (w26:string[])
          }
        }
      }
    }
    frame Error {
    }
  }
  "error out" <- w2
